vi "Cleanup.vi"(8 "error in (no error)":errorcluster, 11 "WebSocket Client in":refnum<class "WebSocket Client.lvclass">) -> (0 "error out":errorcluster, 3 "WebSocket Client out":refnum<class "WebSocket Client.lvclass">)   [LabVIEW 2020, in "HTTP Server.lvlib" / "WebSocket Client.lvclass"]
uses:
  WebSocket Client.lvclass
  WebSocket Client.lvclass/WebSocket Client.ctl
  WebSocket Manager/WebSocket Manager.lvclass
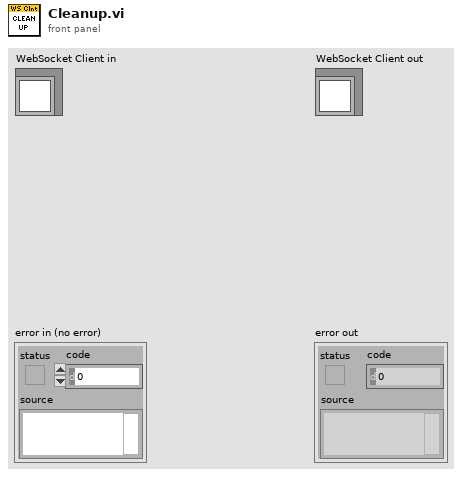
[diagram p1: front panel]
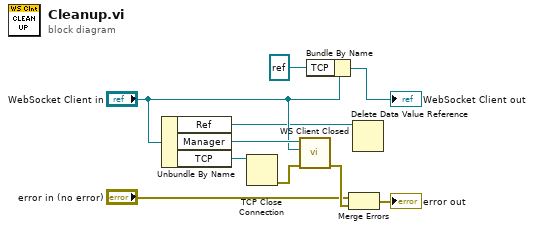
[diagram p0: block diagram]
diagram:
  n1 = Unbundle By Name("WebSocket Client in") -> ("Ref"=w1:refnum<data-value>, "Manager"=w9:refnum<class "WebSocket Manager.lvclass">, "TCP"=w10:refnum<k5>)
  n2 = TCP Close Connection(connection ID=w10) -> (error out=w8:errorcluster)  [unwired: 2 in, 1 out]
  n3 = call-dynamic "WS Client Closed.vi"("error in (no error)"=w8, "WS Client"="WebSocket Client in", "WebSocket Manager in"=w9) -> ("error out"=w7:errorcluster)  [unwired: 8 in]
  n4 = Bundle By Name(cluster="WebSocket Client in", "TCP"=refnum<k5> refnum) -> (→"WebSocket Client out":refnum<class "WebSocket Client.lvclass">)
  n5 = Merge Errors("error in (no error)", w7) -> (→"error out":errorcluster)
  n6 = Delete Data Value Reference(data value reference=w1) -> ()  [unwired: 1 in, 2 out]
